vi "Laser 1 Operations L2 (direct).vi"(0 "Ls1 Visa \nresource":T2, 1 "Laser Ops\n actions":T3, 2 "Ls Data":string[](array[string]), 3 "UI elements cluster":T1, 5 "PreChrp1 \nVisa resource":T2, 9 "Wavelength \n(set) [nm]":u16, 11 "error in (no error)":errorcluster, 12 "Boolean I/P":bool) -> (4 "Ls Data":string[](array[string]), 6 "Resp Validated":bool, 10 "Resp Validated (array) ?":bool[](array[boolean]), 13 "prism Values":dbl[](array[numeric]), 14 "Ls Response":string[](array[string]), 15 "error out":errorcluster)   [LabVIEW 2020]
uses:
  Type Defs/Ls1 Operations.ctl
  Serial Comms/Visa resource.ctl
  Typedefs/UI ctrl refs cluster.ctl
  Typedefs/Laser control knob.ctl
  Typedefs/Frame Size.ctl
  Typedefs/Plane Mode.ctl
  Typedefs/PMT control knob.ctl
  Typedefs/XY Stage_Move.ctl
  Typedefs/test_fpga_control.ctl
  Acquisition/Typedefs/Ref DAQ Param.ctl
  User Interface/Misc/Experiment Type.ctl
  User Interface/Misc/Biology Information.ctl
  Coherent Control/Type defs/Coherent comms control.ctl
  Coherent Control/Type defs/Coherent commands direct mode.ctl
  Coherent Control/Type defs/Commands List.ctl
  Prechirper control/Prechirper commands.ctl
  Typedefs/fgv_actions.ctl
panel:
  in  "prism Values":dbl[](array[numeric])
  # "{True = Open, False = closed}"
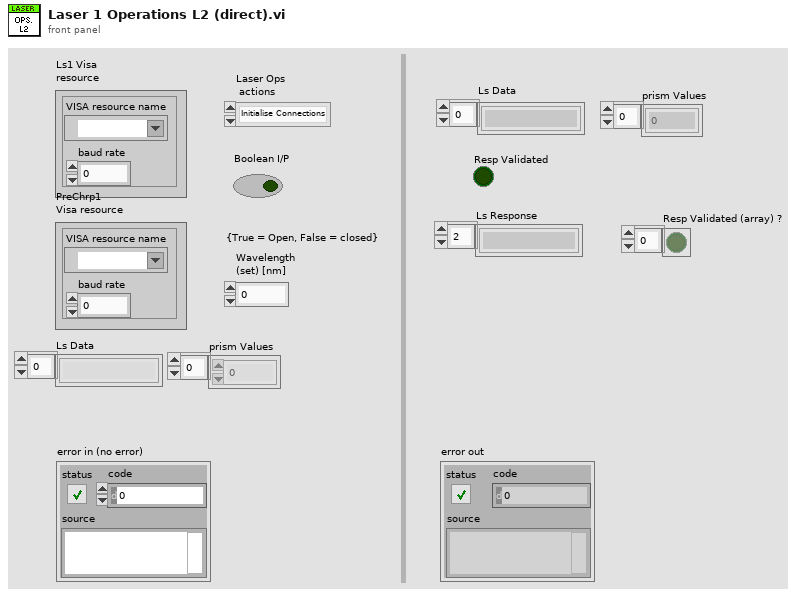
[diagram p1: front panel]
types:
  T1 = typedef "UI ctrl refs cluster.ctl" = cluster{"Top level VI path":path, "Top level VI ref":refnum<vi>, "User menu ref":refnum<k9>, "Sub Panel control":refnum<vi>, "Imaging Param Tab":refnum<vi>, "Occurrence-Start drivers":refnum<k4>, "Occurrence-Speed logging initialised":refnum<k4>, "Occurrence-XYZ stage initialised":refnum<k4>, "Exit button":refnum<vi>, "Status ind":refnum<vi>, "Set as origin":refnum<vi>, "Speed Logging":refnum<vi>, "Time Lapse":refnum<vi>, "Live Imaging":refnum<vi>, "AOL Z Stack":refnum<vi>, "Motor Z Stack":refnum<vi>, "Funct Acq button":refnum<vi>, "Hard Shutter":refnum<vi>, "Virtual Shutter":refnum<vi>, "Laser Power":refnum<vi>, "AOL Mode":refnum<vi>, "Frame Size":refnum<vi>, "Field of View":refnum<vi>, "Dwell Time":refnum<vi>, "Zoom":refnum<vi>, "AOL Z":refnum<vi>, "Objective":refnum<vi>, "Axis":refnum<vi>, "Paths & Names":refnum<vi>, "Experiment folder path (ind.)":refnum<vi>, "Last State (Ind.)":refnum<vi>, "Averages":refnum<vi>, "Angle (degrees)":refnum<vi>, "X centre":refnum<vi>, "Y centre":refnum<vi>, "Plane Mode":refnum<vi>, "# Planes":refnum<vi>, "Z Start":refnum<vi>, "Z Stop":refnum<vi>, "Z Step":refnum<vi>, "PMT 1":refnum<vi>, "PMT 2":refnum<vi>, "Stage XYZ Position":refnum<vi>, "Pockels@Z Start":refnum<vi>, "Pockels@Z Stop":refnum<vi>, "Obtain Z Start":refnum<vi>, "Obtain Z Stop":refnum<vi>, "Live stim.trig.period":refnum<vi>, "Live stim.trig.enable":refnum<vi>, "Movement Correction":refnum<vi>, "Load Reference Image":refnum<vi>, "XY Stage Move":refnum<vi>, "MovCor Cluster":refnum<vi>, "RefDAQParam":refnum<vi>, "Funct. Acq. Pockels Modulation":refnum<vi>, "Ref Laser Power":refnum<vi>, "Enable Video Recording":refnum<vi>, "Video Record-Live Imaging":refnum<vi>, "Video Record-Funct acq":refnum<vi>, "Reference Source":refnum<vi>, "AOL Z-stack Chirps Ready (ind)":refnum<vi>, "Target time between mov.cor. ref triggers (ms)":refnum<vi>, "Funct. Acq. Ref frame save":refnum<vi>, "Tracking button":refnum<vi>, "Show ref plots window":refnum<vi>, "Center freq ind (nm)":refnum<vi>, "Pickup mode (ind)":refnum<vi>, "Logging queue (ind)":refnum<vi>, "Back aperture power (ind.)":refnum<vi>, "Power after objective (ind.)":refnum<vi>, "Switch user":refnum<vi>, "Ls1 Conn. Status":refnum<vi>, "Ls1Tuning Status":refnum<vi>, "Ls1 Faults":refnum<vi>, "Ls1 Connection":refnum<vi>, "Ls1 Mode":refnum<vi>, "Ls1 POWER [mW]":refnum<vi>, "Ls1Shutter":refnum<vi>, "Ls1 Wavelength":refnum<vi>, "Ls1 Note":refnum<vi>, "Ls1 Confirm Wav":refnum<vi>, "Ls1 PreChrp Prism1":refnum<vi>, "Ls1 PreChrp Prism2":refnum<vi>, "Ls1 wav top Ind":refnum<vi>, "Ls1 power top Ind":refnum<vi>, "Ls1 Pump peak Hold":refnum<vi>, "Ls1 Status Ind":refnum<vi>, "Ls1 wav cancel":refnum<vi>, "Experiment Type":refnum<vi>, "Biology Information":refnum<vi>, "Camera recording status":refnum<vi>, "Optimise Obj. Pos.":refnum<vi>}
  T2 = typedef "Visa resource.ctl" = cluster{"VISA resource name":refnum<visa-resource-name>, "baud rate":u32}
  T3 = typedef "Ls1 Operations.ctl" = enum16{"Initialise Connections", "Initialise system", "Check Status", "Open/Close Shutter", "Start/Stop Pump Peak Hold", "Set wavelength", "Close"}
  T4 = typedef "Coherent comms control.ctl" = enum16{"Initialise", "Get Command", "Set Command", "Clear Buffer", "Close"}
  T5 = typedef "Coherent commands direct mode.ctl" = cluster{"Commands & Queries":T6, "Data String":string}
  T6 = typedef "Commands List.ctl" = enum16{"E", "B", "FL", "HM", "L", "LBOH", "LBOOPT", "LFP", "PROMPT", "SM", "S", "VW", "VWS", "HB", "HBR", "REQ", "ALIGN", "K", "F", "FH", "UF", "PHLDC", "PZTMC", "PZTXC", "PZTYC", "PHLDP", "PZTMP", "PZTXP", "PZTYP", "PTRK", "MDLK", "PP", "TS", "STPRPOS", "C", "D1C", "D2C", "BT", "D1T", "D2T", "VT", "LBOT", "ET", "D1ST", "D2ST", "VST", "LBOST", "EST", "D1TD", "D2TD", "VD", "LBOD", "ED", "D1HST", "D2HST", "LRS", "D1SS", "D2SS", "VSS", "LBOSS", "ESS", "D1H", "D2H", "HH", "D1V", "D2V", "SV", "MB", "PI", "BV", "AMDLK", "PZTS", "TMAX", "TMIN", "ALIGNP", "ALIGNW", "PZTXCM", "PZTXCP", "PZTXPM", "PZTXPP", "PZTYCM", "PZTYCP", "PZTYPM", "PZTYPP", "RH", "SN", "ST", "GDDCURVE", "GDD", "GDDCURVEN", "SETCURVEN", "SETCURVEPT", "SAVECURVE", "DELCURVE", "CURVEN", "CURVEPT", "CURVE", "COMP", "HMCOMP", "GDDMAX", "GDDMIN"}
  T7 = typedef "fgv_actions.ctl" = enum16{"Get", "Set"}
  T8 = typedef "Prechirper commands.ctl" = enum16{"Prism 1 read", "Prism 1 set", "Prism 2 read", "Prism 2 set", "Wavelength read", "Wavelength Femto set", "Wavelength Femto and Laser set", "GVD curve number read", "GVD curve number set"}
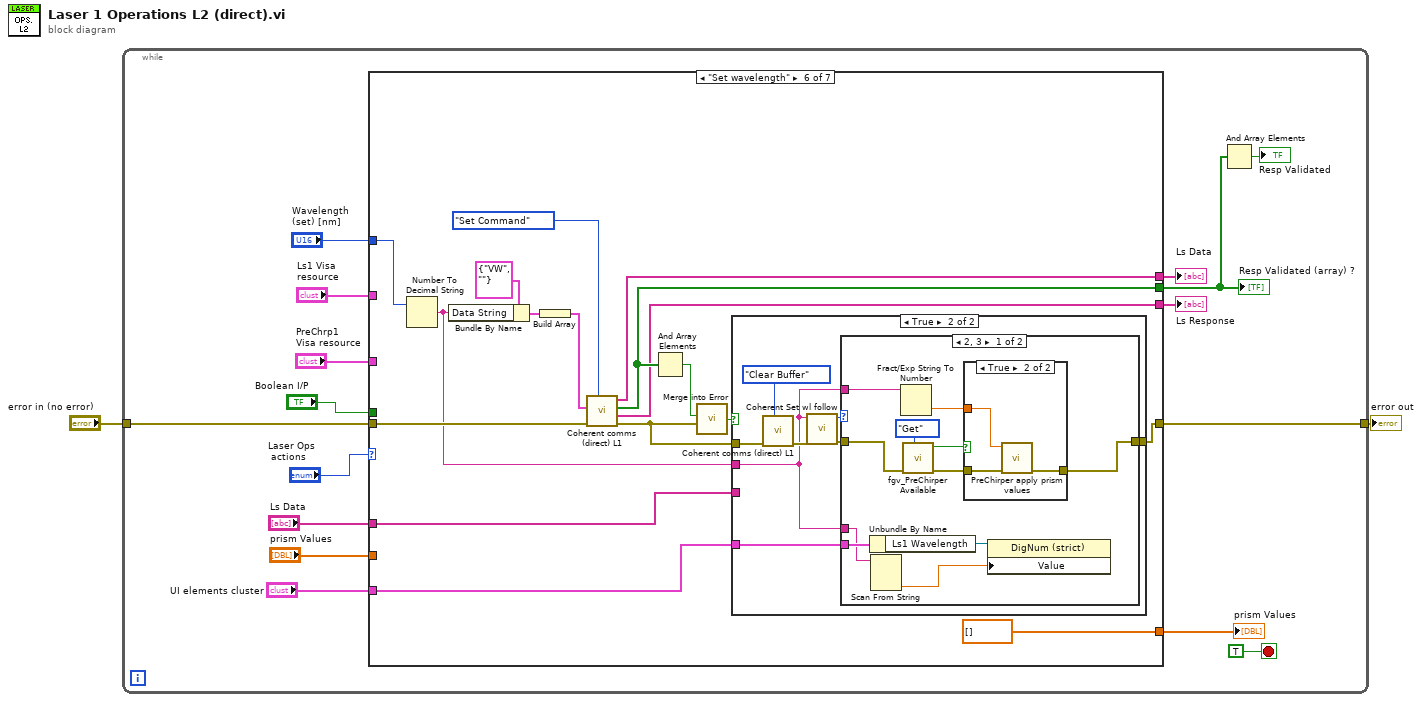
[diagram p0: block diagram]
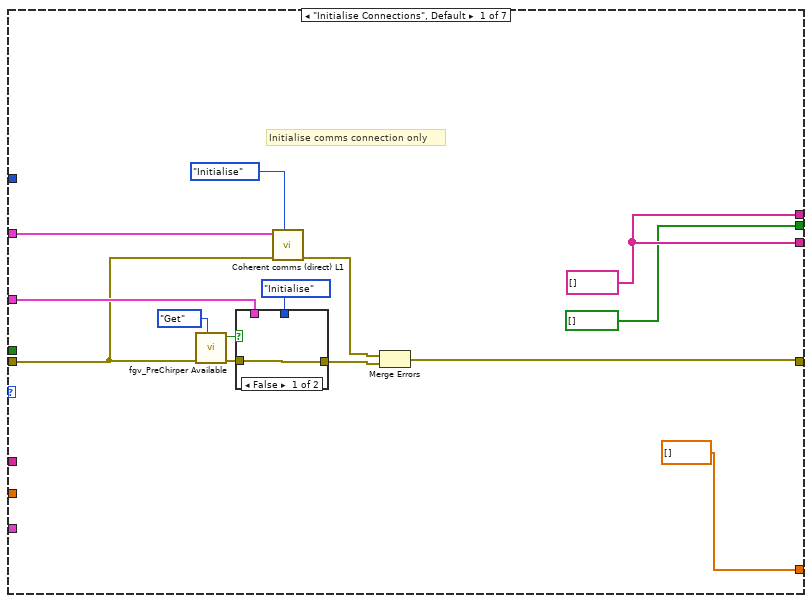
[diagram p2: hidden frame]
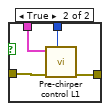
[diagram p3: hidden frame]
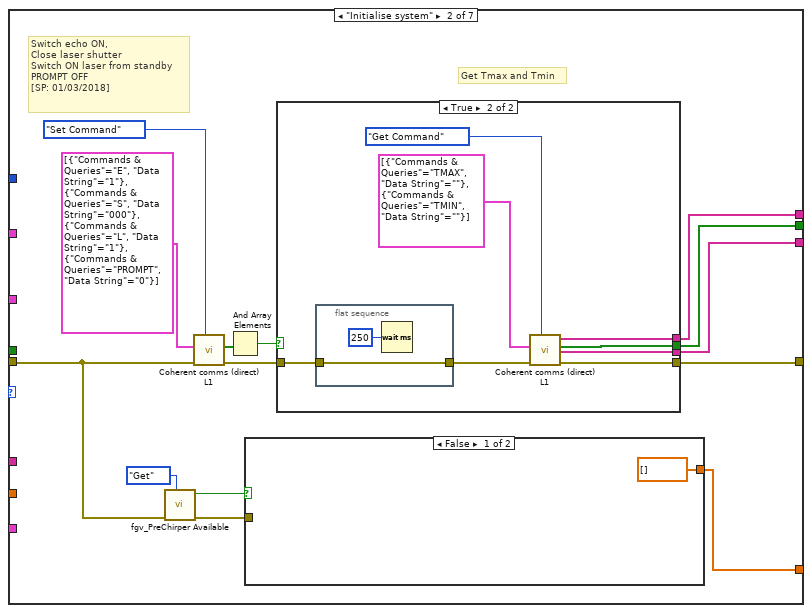
[diagram p4: hidden frame]
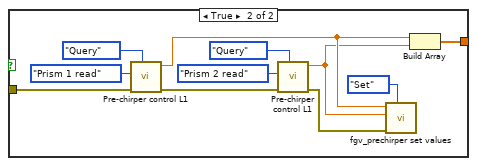
[diagram p5: hidden frame]
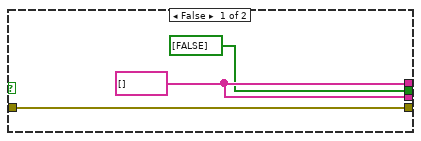
[diagram p6: hidden frame]
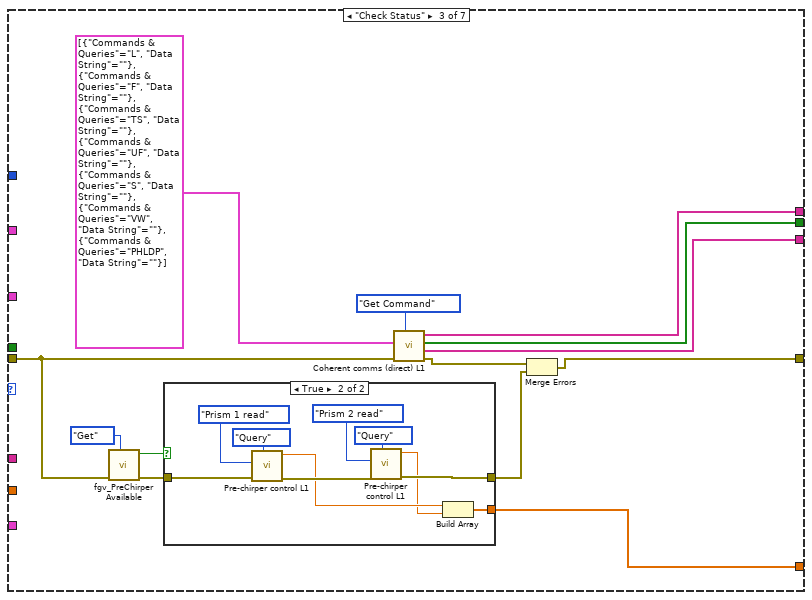
[diagram p7: hidden frame]
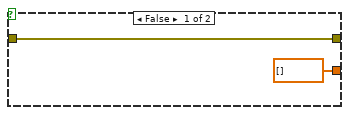
[diagram p8: hidden frame]
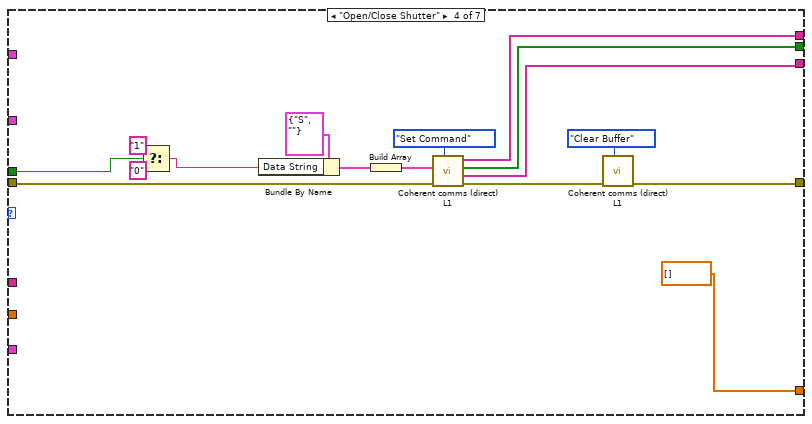
[diagram p9: hidden frame]
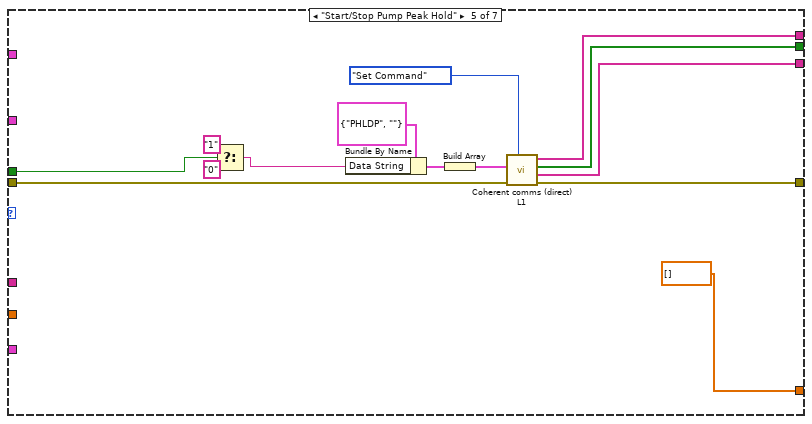
[diagram p10: hidden frame]
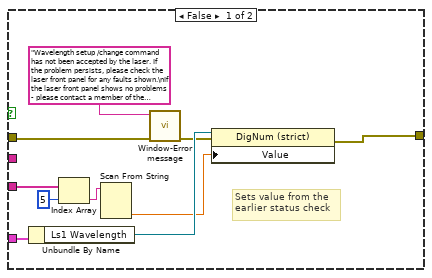
[diagram p11: hidden frame]
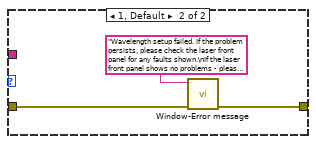
[diagram p13: hidden frame]
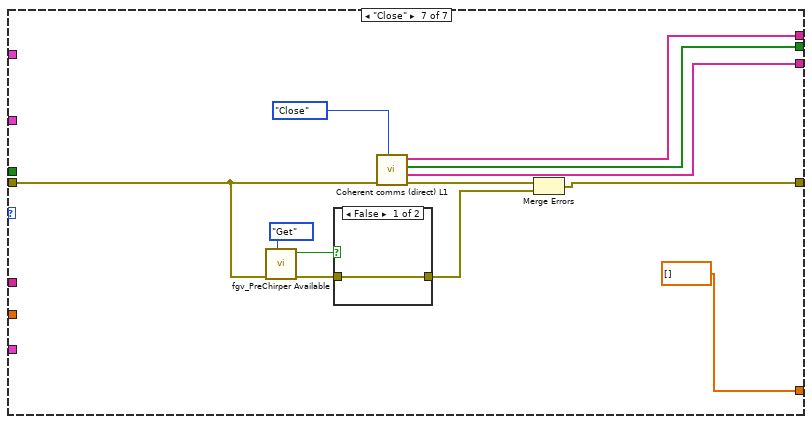
[diagram p14: hidden frame]
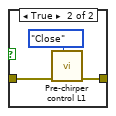
[diagram p15: hidden frame]
diagram:
  n1 = while {
    tunnel: "error in (no error)" -> [w17]
    tunnel: [w16] -> w1
    stop <- TRUE stop-if-true
    n2 = case shown="\"Set wavelength\"" "Laser Ops\n actions" {
      tunnel: w17 -> [w21 w41 w82 w117 w130 w136 w189]
      tunnel: [w28 w49 w79 w102 w131 w142 w186] -> w16
      tunnel: [w27 w48 w88 w109 w123 w144 w196] -> w14
      tunnel: [bool[] [] ("Resp Validated ?") w46 w87 w108 w122 w143 w195] -> w10
      tunnel: [w27 w47 w86 w107 w121 w138 w194] -> w13
      tunnel: "Boolean I/P" -> [_ _ _ w106 w120 _ _]
      tunnel: "Wavelength \n(set) [nm]" -> [_ _ _ _ _ w148 _]
      tunnel: "Ls1 Visa \nresource" -> [w25 _ _ _ _ _ _]
      tunnel: "PreChrp1 \nVisa resource" -> [w24 _ _ _ _ _ _]
      tunnel: [dbl[] [] w43 w78 dbl[] [] dbl[] [] dbl[] [] dbl[] []] -> w6
      tunnel: "Ls Data" -> [_ _ _ _ _ w133 _]
      tunnel: "prism Values" -> [_ _ _ _ _ _ _]
      tunnel: "UI elements cluster" -> [_ _ _ _ _ w132 _]
      frame "Initialise Connections", Default {
        w27 = string[] [] ("Data")
        # "Initialise comms connection only"
        n3 = call "fgv_PreChirper Available.vi"("FGV Actions"=enum16{"Get", "Set"}."Get", "error in (no error)"=w21) -> ("error out"=w20:errorcluster, "PreChirper Available ? OUT"=w23:bool)  [unwired: 8 in]
        n4 = case shown="False" w23 {
          tunnel: enum16{"Initialise", "Query", "Close"}."Initialise" ("State") -> [_ w37]
          tunnel: w20 -> [w33 w36]
          tunnel: [w33 w35] -> w30
          tunnel: w24 -> [_ w34]
          frame False {
          }
          frame True {
            n5 = call "Pre-chirper control L1.vi"("State"=w37, "error in (no error)"=w36, "Visa resource"=w34) -> ("error out"=w35:errorcluster)  [unwired: 7 in, 1 out]
          }
        }
        n6 = call "Coherent comms (direct) L1.vi"("Coherent laser commands L1"=Coherent_comms_control."Initialise", "error in (no error)"=w21, "Visa resource"=w25) -> ("error out"=w29:errorcluster)  [unwired: 4 in, 4 out]
        n7 = Merge Errors(w29, w30) -> (w28:errorcluster)
      }
      frame "Initialise system" {
        # "Switch echo ON,\nClose laser shutter\nSwitch ON laser from standby\nPROMPT OFF\n[SP: 01/03/2018]"
        # "Get Tmax and Tmin"
        n8 = call "fgv_PreChirper Available.vi"("FGV Actions"=enum16{"Get", "Set"}."Get", "error in (no error)"=w41) -> ("error out"=w40:errorcluster, "PreChirper Available ? OUT"=w39:bool)  [unwired: 8 in]
        n9 = call "Coherent comms (direct) L1.vi"("Coherent laser commands L1"=Coherent_comms_control."Set Command", "error in (no error)"=w41, "Commands \nand Queries"=T5[] [{"Commands & Queries"=enum."E", "Data String"="1"}, {"Commands & Queries"=enum."S", "Data String"="000"}, {"Commands & Queries"=enum."L", "Data String"="1"}, {"Commands & Queries"=enum."PROMPT", "Data String"="0"}] ("Commands \nand Queries")) -> ("error out"=w50:errorcluster, "Resp Validated ?"=w45:bool[])  [unwired: 4 in, 3 out]
        n10 = And Array Elements(Boolean array=w45) -> (logical AND=w44:bool)
        n11 = case shown="False" w39 {
          tunnel: w40 -> [_ w63]
          tunnel: [dbl[] [] w53] -> w43
          frame False {
          }
          frame True {
            n12 = call "Pre-chirper control L1.vi"("State"=enum16{"Initialise", "Query", "Close"}."Query", "error in (no error)"=w63, "Pre-chirper commands"=Prechirper_commands."Prism 1 read") -> ("error out"=w58:errorcluster, "number"=w55:dbl)  [unwired: 7 in]
            n13 = call "Pre-chirper control L1.vi"("State"=enum16{"Initialise", "Query", "Close"}."Query", "error in (no error)"=w58, "Pre-chirper commands"=Prechirper_commands."Prism 2 read") -> ("error out"=w56:errorcluster, "number"=w54:dbl)  [unwired: 7 in]
            n14 = call "fgv_prechirper set values.vi"("FGV Actions"=fgv_actions."Set", "error in (no error)"=w56, "Prism A value [IN]"=w54, "Prism B value [IN]"=w55) -> ()  [unwired: 5 in, 3 out]
            n15 = Build Array(w55, w54) -> (w53:dbl[])
          }
        }
        n16 = case shown="True" w44 {
          tunnel: w50 -> [w66 w69]
          tunnel: [w66 w71] -> w49
          tunnel: [w65 w70] -> w48
          tunnel: [w65 w73] -> w47
          tunnel: [bool[] [FALSE] ("Resp Validated ?") w72] -> w46
          frame False {
            w65 = string[] [] ("Data")
          }
          frame True {
            n17 = flat-sequence {
              tunnel: w69 -> [w76]
              tunnel: [w76] -> w68
              frame #0 {
                n18 = Wait (ms)(milliseconds to wait=u32 250) -> ()  [unwired: 1 out]
              }
            }
            n19 = call "Coherent comms (direct) L1.vi"("Coherent laser commands L1"=Coherent_comms_control."Get Command", "error in (no error)"=w68, "Commands \nand Queries"=T5[] [{"Commands & Queries"=enum."TMAX", "Data String"=""}, {"Commands & Queries"=enum."TMIN", "Data String"=""}] ("Commands \nand Queries")) -> ("error out"=w71:errorcluster, "Response"=w73:string[], "Resp Validated ?"=w72:bool[], "Data"=w70:string[])  [unwired: 4 in, 1 out]
          }
        }
      }
      frame "Check Status" {
        n20 = call "fgv_PreChirper Available.vi"("FGV Actions"=enum16{"Get", "Set"}."Get", "error in (no error)"=w82) -> ("error out"=w83:errorcluster, "PreChirper Available ? OUT"=w85:bool)  [unwired: 8 in]
        n21 = case shown="True" w85 {
          tunnel: w83 -> [w91 w101]
          tunnel: [w91 w98] -> w80
          tunnel: [dbl[] [] w92] -> w78
          frame False {
          }
          frame True {
            n22 = call "Pre-chirper control L1.vi"("State"=enum16{"Initialise", "Query", "Close"}."Query", "error in (no error)"=w101, "Pre-chirper commands"=Prechirper_commands."Prism 1 read") -> ("error out"=w99:errorcluster, "number"=w94:dbl)  [unwired: 7 in]
            n23 = call "Pre-chirper control L1.vi"("State"=enum16{"Initialise", "Query", "Close"}."Query", "error in (no error)"=w99, "Pre-chirper commands"=Prechirper_commands."Prism 2 read") -> ("error out"=w98:errorcluster, "number"=w93:dbl)  [unwired: 7 in]
            n24 = Build Array(w94, w93) -> (w92:dbl[])
          }
        }
        n25 = call "Coherent comms (direct) L1.vi"("Coherent laser commands L1"=Coherent_comms_control."Get Command", "error in (no error)"=w82, "Commands \nand Queries"=T5[] [{"Commands & Queries"=enum."L", "Data String"=""}, {"Commands & Queries"=enum."F", "Data String"=""}, {"Commands & Queries"=enum."TS", "Data String"=""}, {"Commands & Queries"=enum."UF", "Data String"=""}, {"Commands & Queries"=enum."S", "Data String"=""}, {"Commands & Queries"=enum."VW", "Data String"=""}, {"Commands & Queries"=enum."PHLDP", "Data String"=""}] ("Commands \nand Queries")) -> ("error out"=w81:errorcluster, "Response"=w86:string[], "Resp Validated ?"=w87:bool[], "Data"=w88:string[])  [unwired: 4 in, 1 out]
        n26 = Merge Errors(w81, w80) -> (w79:errorcluster)
      }
      frame "Open/Close Shutter" {
        n27 = Select(t="1" ("Data String"), s=w106, f="0" ("Data String")) -> (s? t:f=w113:string)
        n28 = Bundle By Name(cluster=T5 {"Commands & Queries"=enum."S", "Data String"=""} ("Coherent Commands"), "Data String"=w113) -> (w111:T5)
        n29 = Build Array(w111) -> (w112:T5[])
        n30 = call "Coherent comms (direct) L1.vi"("Coherent laser commands L1"=Coherent_comms_control."Set Command", "error in (no error)"=w117, "Commands \nand Queries"=w112) -> ("error out"=w103:errorcluster, "Response"=w107:string[], "Resp Validated ?"=w108:bool[], "Data"=w109:string[])  [unwired: 4 in, 1 out]
        n31 = call "Coherent comms (direct) L1.vi"("Coherent laser commands L1"=Coherent_comms_control."Clear Buffer", "error in (no error)"=w103) -> ("error out"=w102:errorcluster)  [unwired: 5 in, 4 out]
      }
      frame "Start/Stop Pump Peak Hold" {
        n32 = Select(t="1" ("Data String"), s=w120, f="0" ("Data String")) -> (s? t:f=w126:string)
        n33 = Bundle By Name(cluster=T5 {"Commands & Queries"=enum."PHLDP", "Data String"=""} ("Coherent Commands"), "Data String"=w126) -> (w124:T5)
        n34 = Build Array(w124) -> (w125:T5[])
        n35 = call "Coherent comms (direct) L1.vi"("Coherent laser commands L1"=Coherent_comms_control."Set Command", "error in (no error)"=w130, "Commands \nand Queries"=w125) -> ("error out"=w131:errorcluster, "Response"=w121:string[], "Resp Validated ?"=w122:bool[], "Data"=w123:string[])  [unwired: 4 in, 1 out]
      }
      frame "Set wavelength" {
        n36 = Number To Decimal String(number=w148) -> (decimal integer string=w135:string)  [unwired: 1 in]
        n37 = Bundle By Name(cluster=T5 {"Commands & Queries"=enum."VW", "Data String"=""} ("Coherent Commands"), "Data String"=w135) -> (w145:T5)
        n38 = Build Array(w145) -> (w146:T5[])
        n39 = call "Coherent comms (direct) L1.vi"("Coherent laser commands L1"=Coherent_comms_control."Set Command", "error in (no error)"=w136, "Commands \nand Queries"=w146) -> ("error out"=w140:errorcluster, "Response"=w138:string[], "Resp Validated ?"=w143:bool[], "Data"=w144:string[])  [unwired: 4 in, 1 out]
        n40 = And Array Elements(Boolean array=w143) -> (logical AND=w141:bool)
        n41 = call "Merge into Error.vi"("Boolean in"=w141, "error in (no error)"=w140) -> ("Boolean out"=w139:bool)  [unwired: 6 in]
        n42 = case shown="True" w139 {
          tunnel: w140 -> [w158 w162]
          tunnel: [w151 w165] -> w142
          tunnel: w135 -> [_ w160]
          tunnel: w133 -> [w156 _]
          tunnel: w132 -> [w154 w159]
          frame False {
            # "Sets value from the \nearlier status check"
            n43 = Unbundle By Name(w154) -> ("Ls1 Wavelength"=w153:refnum<vi>)
            n44 = Index Array(array=w156, index=5) -> (element=w150:string)
            n45 = Scan From String(input string=w150) -> (output 1=w149:dbl)  [unwired: 4 in, 3 out]
            n46 = call "Window-Error message.vi"("error in (no error)"=w158, "Message"="Wavelength setup /change command has not been accepted by the laser. If the problem persists, please check the laser front panel for any faults shown.\nIf the laser front panel shows no problems - please contact a member of the microscope team.") -> ("Error Out (no error)"=w152:errorcluster)  [unwired: 9 in]
            n47 = property class="DigNum (strict)"(reference=w153, error in=w152, "Value"=w149) -> (error out=w151:errorcluster)  [unwired: 1 out]
          }
          frame True {
            n48 = call "Coherent comms (direct) L1.vi"("Coherent laser commands L1"=Coherent_comms_control."Clear Buffer", "error in (no error)"=w162) -> ("error out"=w161:errorcluster)  [unwired: 5 in, 4 out]
            n49 = call "Coherent Set wl follow.vi"("error in (no error)"=w161, "Wavelength"=w160) -> ("error out"=w166:errorcluster, "exit code"=w164:u32)  [unwired: 8 in]
            n50 = case shown="2, 3" w164 {
              tunnel: w166 -> [w175 w184]
              tunnel: [w172 w183] -> w165
              tunnel: w160 -> [w177 _]
              tunnel: w160 -> [w168 _]
              tunnel: w159 -> [w170 _]
              frame 2, 3 {
                n51 = Unbundle By Name(w170) -> ("Ls1 Wavelength"=w169:refnum<vi>)
                n52 = Scan From String(input string=w168) -> (output 1=w167:dbl)  [unwired: 4 in, 3 out]
                n53 = Fract/Exp String To Number(string=w177) -> (number=w171:dbl)  [unwired: 3 in, 1 out]
                n54 = call "fgv_PreChirper Available.vi"("FGV Actions"=enum16{"Get", "Set"}."Get", "error in (no error)"=w175) -> ("error out"=w173:errorcluster, "PreChirper Available ? OUT"=w174:bool)  [unwired: 8 in]
                n55 = case shown="True" w174 {
                  tunnel: w173 -> [w178 w181]
                  tunnel: [w178 w180] -> w172
                  tunnel: w171 -> [_ w179]
                  frame False {
                  }
                  frame True {
                    n56 = call "PreChirper apply prism values.vi"("error in (no error)"=w181, "Wavelength"=w179) -> ("error out"=w180:errorcluster)  [unwired: 9 in]
                  }
                }
                n57 = property class="DigNum (strict)"(reference=w169, "Value"=w167) -> ()  [unwired: 1 in, 2 out]
              }
              frame 1, Default {
                n58 = call "Window-Error message.vi"("error in (no error)"=w184, "Message"="Wavelength setup failed. If the problem persists, please check the laser front panel for any faults shown.\nIf the laser front panel shows no problems - please contact a member of the microscope team.") -> ("Error Out (no error)"=w183:errorcluster)  [unwired: 9 in]
              }
            }
          }
        }
      }
      frame "Close" {
        n59 = call "fgv_PreChirper Available.vi"("FGV Actions"=enum16{"Get", "Set"}."Get", "error in (no error)"=w189) -> ("error out"=w190:errorcluster, "PreChirper Available ? OUT"=w192:bool)  [unwired: 8 in]
        n60 = case shown="False" w192 {
          tunnel: w190 -> [w197 w200]
          tunnel: [w197 w199] -> w187
          frame False {
          }
          frame True {
            n61 = call "Pre-chirper control L1.vi"("State"=enum16{"Initialise", "Query", "Close"}."Close", "error in (no error)"=w200) -> ("error out"=w199:errorcluster)  [unwired: 8 in, 1 out]
          }
        }
        n62 = call "Coherent comms (direct) L1.vi"("Coherent laser commands L1"=Coherent_comms_control."Close", "error in (no error)"=w189) -> ("error out"=w188:errorcluster, "Response"=w194:string[], "Resp Validated ?"=w195:bool[], "Data"=w196:string[])  [unwired: 5 in, 1 out]
        n63 = Merge Errors(w188, w187) -> (w186:errorcluster)
      }
    }
    "Ls Data" <- w14
    "Resp Validated (array) ?" <- w10
    "Ls Response" <- w13
    "prism Values" <- w6
    n64 = And Array Elements(Boolean array=w10) -> (logical AND=→"Resp Validated":bool)
  }
  "error out" <- w1
